vi "Read Alarm Limits.vi"(8 "error in":errorcluster, 11 "Value in":refnum<class "Value.lvclass">) -> (0 "error out":errorcluster, 1 "has alarm limits?":bool, 2 "alarm limits":T1={"Active"=FALSE, "Low Alarm Limit"=0.0, "Low Warning Limit"=0.0, "High Warning Limit"=0.0, "High Alarm Limit"=0.0, "Low Alarm Severity"=enum."major", "Low Warning Severity"=enum."minor", "High Warning Severity "=enum."minor", "High Alarm Severity"=enum."major", "Hysteresis"=0.0}, 3 "Value out":refnum<class "Value.lvclass">)   [LabVIEW 2020, in "Value.lvlib" / "Value.lvclass"]
uses:
  Value.lvclass
  Value.lvclass/Value.ctl
  Alarm Severity.ctl
  Value.lvlib
  Alarm Limits.ctl
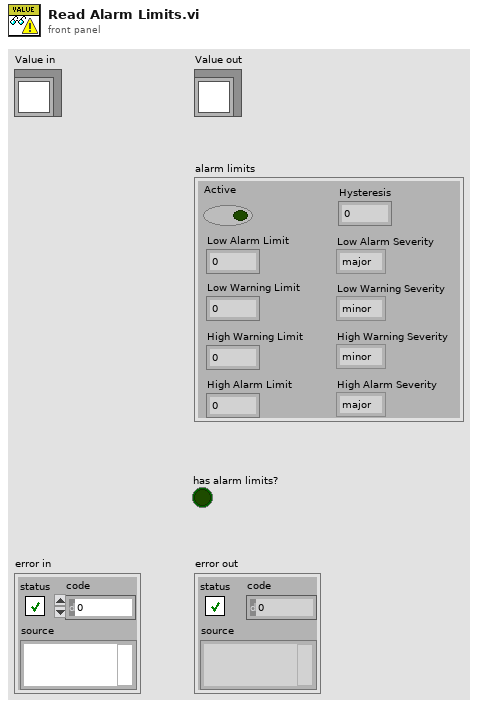
[diagram p1: front panel]
types:
  T1 = typedef "Value.lvlib/Alarm Limits.ctl" = cluster{"Active":bool, "Low Alarm Limit":dbl, "Low Warning Limit":dbl, "High Warning Limit":dbl, "High Alarm Limit":dbl, "Low Alarm Severity":T2, "Low Warning Severity":T2, "High Warning Severity ":T2, "High Alarm Severity":T2, "Hysteresis":dbl}
  T2 = typedef "Value.lvlib/Alarm Severity.ctl" = enum32{"no", "minor", "major", "record", "invalid", "undefined", ""}
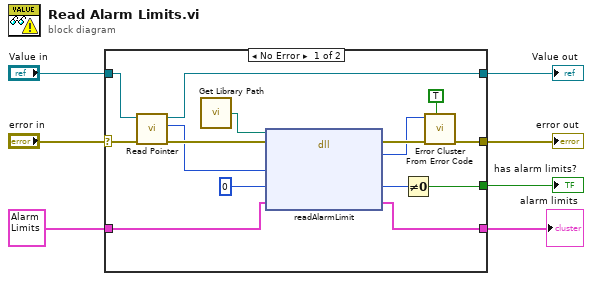
[diagram p0: block diagram]
diagram:
  n1 = case shown="No Error" "error in" {
    selector: "error in" -> [w17 w24]
    tunnel: [w18 w24] -> w7
    tunnel: "Value in" -> [w15 w23]
    tunnel: [w13 w23] -> w4
    tunnel: T1 {"Active"=FALSE, "Low Alarm Limit"=0.0, "Low Warning Limit"=0.0, "High Warning Limit"=0.0, "High Alarm Limit"=0.0, "Low Alarm Severity"=enum."major", "Low Warning Severity"=enum."minor", "High Warning Severity "=enum."minor", "High Alarm Severity"=enum."major", "Hysteresis"=0.0} ("Alarm Limits") -> [w12 _]
    tunnel: [w8 _] -> w3
    tunnel: [w9 _] -> w2
    frame No Error {
      n2 = call-dynamic "Read Pointer.vi"("error in (no error)"=w17, "Value in"=w15) -> ("error out"=w16:errorcluster, "pointer"=w14:i64, "Value out"=w13:refnum<class "Value.lvclass">)  [unwired: 7 in]
      n3 = call "Get Library Path.vi"() -> ("Path"=w22:path)  [unwired: 1 in]
      n4 = dll-call lib="?" fn="readAlarmLimit"(path in=w22, error in=w16, "value"=w14, "has alarm limits?"=i16 0 ("has display metadata?"), "alarm limits"=w12) -> (error out=w20:errorcluster, "err_code"=w19:i32, "has alarm limits?"=w11:i16, "alarm limits"=w9:T1)  [unwired: 2 in, 1 out]
      n5 = Not Equal To 0?(x=w11) -> (x != 0?=w8:bool)
      n6 = call <vilib>:"Error Cluster From Error Code.vi"("show call chain? (False)"=TRUE, "error in (no error)"=w20, "error code (0)"=w19) -> ("error out"=w18:errorcluster)  [unwired: 6 in]
    }
    frame Error {
    }
  }
  "error out" <- w7
  "Value out" <- w4
  "has alarm limits?" <- w3
  "alarm limits" <- w2
